vi "FRCts20_Backend_Request_PD_reform.vi"(7 "Request":T1, 8 "error in (no error)":errorcluster, 11 "rows affected":i32) -> (0 "error out":errorcluster, 3 "data string":string)   [LabVIEW 2014, in "FRCts20_Backend_Engine.lvlib"]
doc: "Returns whether a specific request was updated or deleted successfully"
uses:
  FRCts20_Backend_Engine.lvlib
  FRCts20_Backend_API/FRCts20_Backend_API_Request.ctl
  FRCts20_Backend_API/FRCts20_Backend_API_Status.ctl
  FRCts20_Backend_API/FRCts20_Backend_API.lvlib
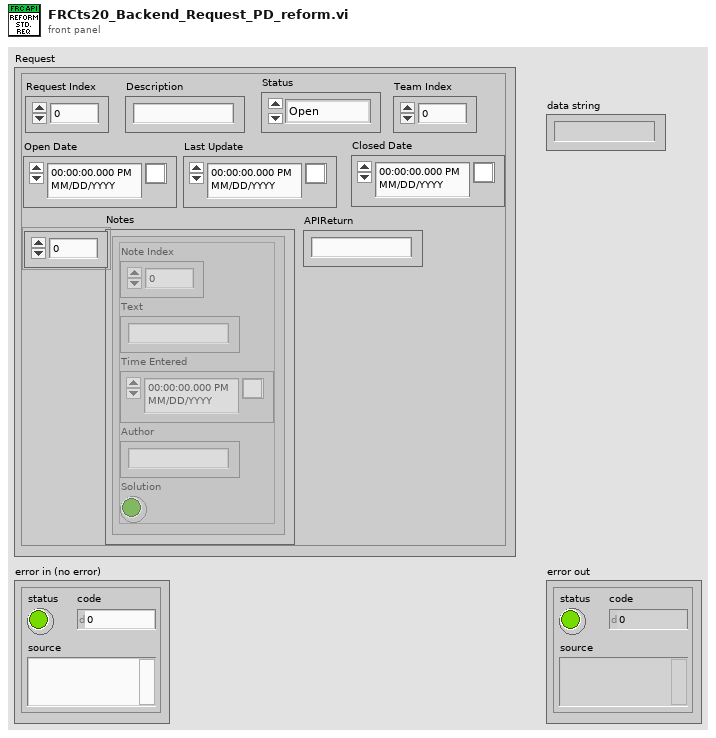
[diagram p1: front panel]
types:
  T1 = typedef "FRCts20_Backend_Engine.lvlib/FRCts20_Backend_API.lvlib/FRCts20_Backend_API_Request.ctl" = cluster{"Request Index":u32, "Description":string, "Status":T2, "Open Date":timestamp, "Last Update":timestamp, "Closed Date":timestamp, "Notes":cluster{"Note Index":u32, "Text":string, "Time Entered":timestamp, "Author":string, "Solution":bool}[], "Team Index":u32, "APIReturn":string}
  T2 = typedef "FRCts20_Backend_Engine.lvlib/FRCts20_Backend_API.lvlib/FRCts20_Backend_API_Status.ctl" = enum16{"Open", "In Work", "Closed"}
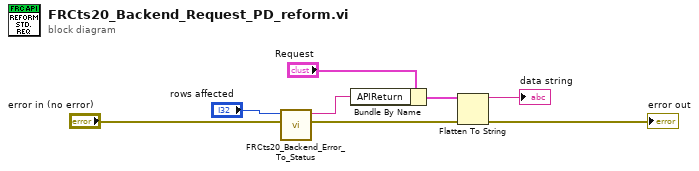
[diagram p0: block diagram]
diagram:
  n1 = call "FRCts20_Backend_Error_To_Status.vi"("error in (no error)"="error in (no error)", "rows affected"="rows affected") -> ("error out"=w6:errorcluster, "String"=w5:string)  [unwired: 8 in]
  n2 = Bundle By Name(cluster="Request", "APIReturn"=w5) -> (w2:T1)
  n3 = Flatten To String(anything=w2, error in (no error)=w6) -> (data string=→"data string":string, error out=→"error out":errorcluster)  [unwired: 2 in, 1 out]
